vi "Setup.vi"(8 "error in (no error)":errorcluster, 9 "Str Refnum":refnum<vi>, 10 "VI Reference":refnum<vi>, 11 "Dialog_TwoButtons in":refnum<class "Dialog_TwoButtons.lvclass">) -> (0 "error out":errorcluster, 2 "VI reference (dup)":refnum<vi>, 3 "Dialog_TwoButtons out":refnum<class "Dialog_TwoButtons.lvclass">)   [LabVIEW 2012, in "Dialog_TwoButtons.lvlib" / "Dialog_TwoButtons.lvclass"]
uses:
  Dialog_TwoButtons.lvclass
  Dialog/Dialog/Dialog.lvclass
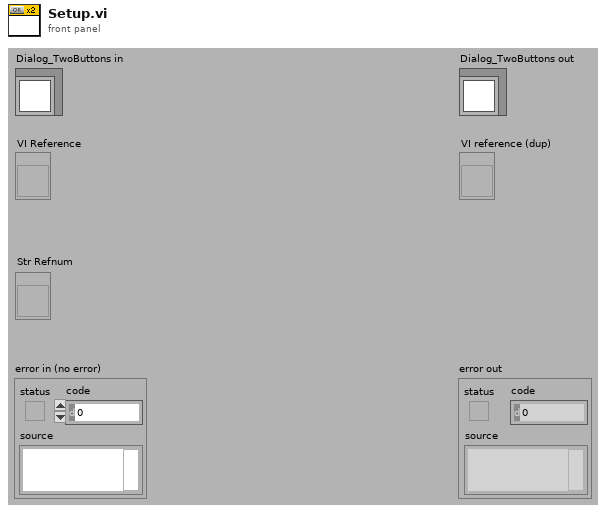
[diagram p1: front panel]
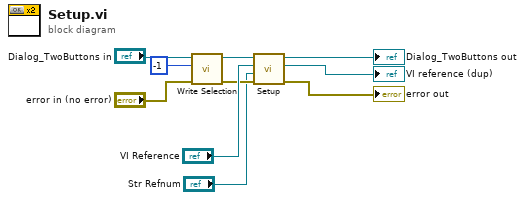
[diagram p0: block diagram]
diagram:
  n1 = call-dynamic "Write Selection.vi"("error in (no error)"="error in (no error)", "Selection (-1: none)"=i8 -1, "Dialog_2Buttons.lvclass in"="Dialog_TwoButtons in") -> ("error out"=w4:errorcluster, "Dialog_2Buttons.lvclass out"=w5:refnum<class "Dialog_TwoButtons.lvclass">)  [unwired: 7 out]
  n2 = call-parent "Setup.vi"("error in (no error)"=w4, "Str Refnum"="Str Refnum", "VI Reference"="VI Reference", "Dialog in"=w5) -> ("error out"=→"error out":errorcluster, "VI reference (dup)"=→"VI reference (dup)":refnum<vi>, "Dialog out"=→"Dialog_TwoButtons out":refnum<class "Dialog_TwoButtons.lvclass">)  [unwired: 5 out]
